vi "ClearArb.vi"(8 "error in (no error)":errorcluster, 10 "Handle":string, 11 "ArbitraryFunction":refnum<class "ArbitraryFunction.lvclass">) -> (0 "error out":errorcluster, 3 "ArbitraryFunction":refnum<class "ArbitraryFunction.lvclass">)   [LabVIEW 2014, in "Functions.lvlib" / "ArbitraryFunction.lvclass"]
uses:
  ArbitraryFunction.lvclass
  ArbitraryFunction.lvclass/ArbitraryFunction.ctl
  Accessors/Read Arbs.vi
  Accessors/Write Arbs.vi
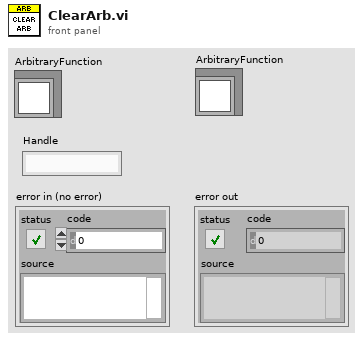
[diagram p1: front panel]
types:
  T1 = typedef "ArbitraryFunction.lvclass/Arbitrary.ctl" = cluster{"Handle":string, "Size":i32, "Gain":dbl, "Offset":dbl, "Waveform":waveform(dbl)}
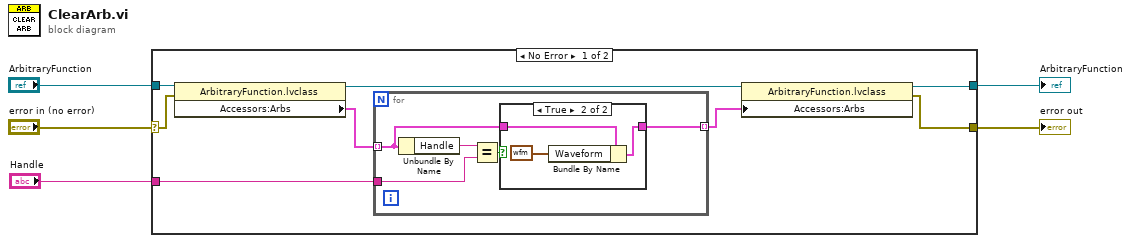
[diagram p0: block diagram]
diagram:
  n1 = case shown="No Error" "error in (no error)" {
    selector: "error in (no error)" -> [w12 w24]
    tunnel: [w6 w24] -> w4
    tunnel: "ArbitraryFunction" -> [w13 w23]
    tunnel: [w7 w23] -> w2
    tunnel: "Handle" -> [w10 _]
    frame No Error {
      n2 = property class="ArbitraryFunction.lvclass"(reference=w13, error in=w12) -> (reference out=w9:refnum<class "ArbitraryFunction.lvclass">, "Accessors:Arbs"=w11:T1[])  [unwired: 1 out]
      n3 = for {
        tunnel: w11 -> [w15] mode=indexing
        tunnel: w10 -> [w17]
        tunnel: [w14] -> w8 mode=indexing
        n4 = Unbundle By Name(w15) -> ("Handle"=w18:string)
        n5 = Equal?(x=w18, y=w17) -> (x = y?=w16:bool)
        n6 = case shown="True" w16 {
          tunnel: w15 -> [w19 w22]
          tunnel: [w19 w20] -> w14
          frame False {
          }
          frame True {
            n7 = Bundle By Name(cluster=w22, "Waveform"=waveform(dbl) {"t0"=timestamp(0 s since 1904-01-01), "dt"=1.0, "Y"=[]}) -> (w20:T1)
          }
        }
      }
      n8 = property class="ArbitraryFunction.lvclass"(reference=w9, "Accessors:Arbs"=w8) -> (reference out=w7:refnum<class "ArbitraryFunction.lvclass">, error out=w6:errorcluster)  [unwired: 1 in]
    }
    frame Error {
    }
  }
  "ArbitraryFunction" <- w2
  "error out" <- w4
